vi "Adressen Filtern.vi"(8 "error in (no error)":errorcluster caption="Fehler (Eingang, kein Fehler)", 10 "AdressIndex":T1, 11 "Steuerung PNS Eingang":refnum<class "Steuerung PNS.lvclass">) -> (0 "error out":errorcluster caption="Fehler (Ausgang)", 2 "Adressen":cluster{i32[][], i32}, 3 "Steuerung PNS Ausgang":refnum<class "Steuerung PNS.lvclass">)   [LabVIEW 2020, in "Steuerung PNS.lvclass"]
uses:
  Steuerung PNS.lvclass
  AdressIndex.ctl
  Steuerung PNS.lvclass/Steuerung PNS.ctl
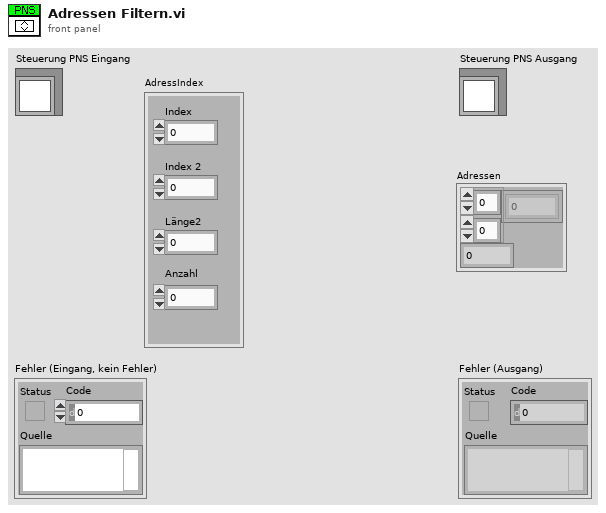
[diagram p1: front panel]
types:
  T1 = typedef "Steuerung PNS.lvclass/AdressIndex.ctl" = cluster{"Index":i32, "Index 2":i32, "Länge2":i32, "\nAnzahl":i32}
  T2 = typedef "Steuerung PNS.lvclass/Adresse.ctl" = cluster{i32[][], i32}
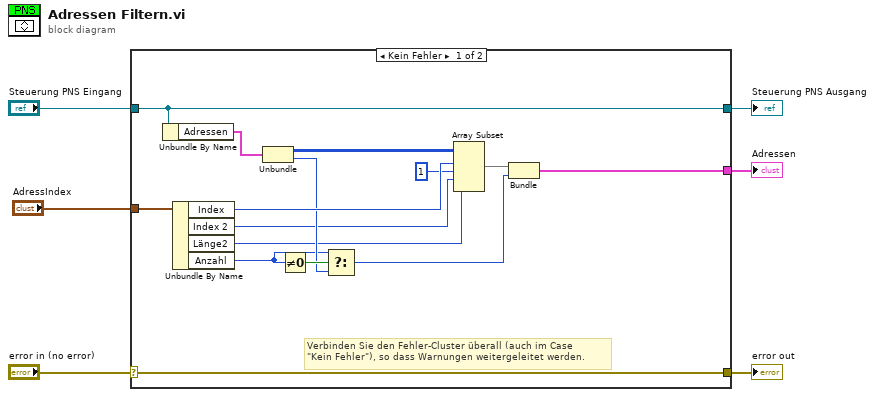
[diagram p0: block diagram]
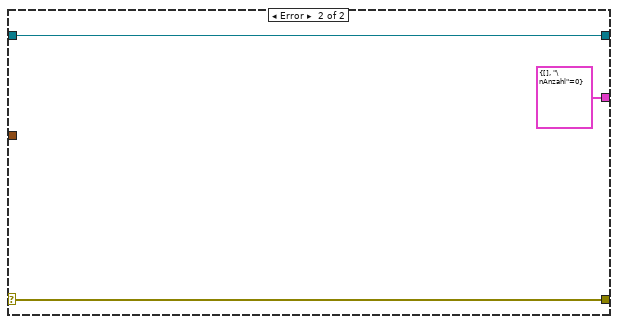
[diagram p2: hidden frame]
diagram:
  n1 = case shown="Kein Fehler" "error in (no error)" {
    selector: "error in (no error)" -> [w21 w24]
    tunnel: [w21 w24] -> w5
    tunnel: [w20 w23] -> w3
    tunnel: "Steuerung PNS Eingang" -> [w20 w23]
    tunnel: "AdressIndex" -> [w19 _]
    tunnel: [w7 cluster{i32[][], "\nAnzahl":i32} {[], "\nAnzahl"=0}] -> w1
    frame No Error {
      # "Verbinden Sie den Fehler-Cluster überall (auch im Case\n\"Kein Fehler\"), so dass Warnungen weitergeleitet werden."
      n2 = Unbundle By Name(w20) -> ("Adressen"=w18:T2)
      n3 = Unbundle By Name(w19) -> ("Index"=w15:i32, "Index 2"=w9:i32, "Länge2"=w8:i32, "Anzahl"=w13:i32)
      n4 = Unbundle(w18) -> (w16:i32[][], w14:i32)
      n5 = Not Equal To 0?(x=w13) -> (x != 0?=w17:bool)
      n6 = Select(t=w13, s=w17, f=w14) -> (s? t:f=w11:i32)
      n7 = Array Subset(array=w16, index (row)=w15, length (row)=1 ("Länge"), index (col)=w9, length (col)=w8) -> (w12:i32[][])
      n8 = Bundle(w12, "Anzahl"=w11) -> (w7:cluster{i32[][], "\nAnzahl":i32})  [unwired: 1 in]
    }
    frame Error {
    }
  }
  "error out" <- w5
  "Steuerung PNS Ausgang" <- w3
  "Adressen" <- w1
